vi "Apply Read Write BitField Mask.vi"(8 "error in":errorcluster, 10 "mask":enum16{"Disable", "Enable"}(ring), 11 "bitfields in":u32 format="%.0b") -> (0 "error out":errorcluster, 3 "bitfields out":u32 format="%.0b")   [LabVIEW 2020, in "Routing and Faulting Scripting.lvlib"]
uses:
  Routing and Faulting Scripting.lvlib
  NationalInstruments.VeriStand.SystemDefinitionAPI
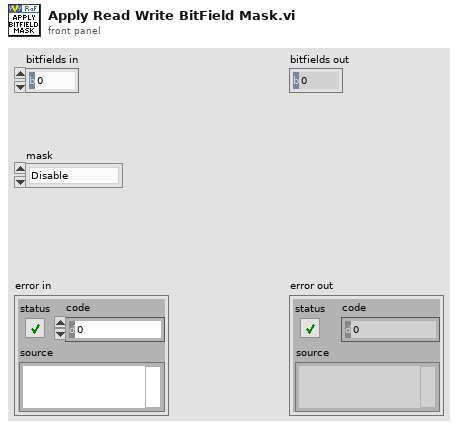
[diagram p1: front panel]
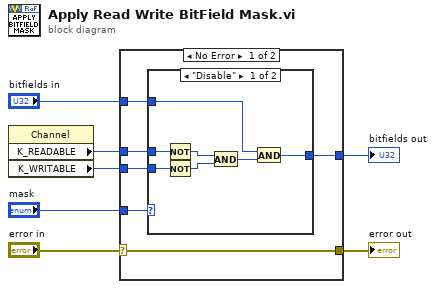
[diagram p0: block diagram]
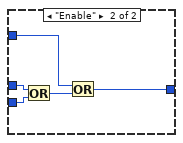
[diagram p2: hidden frame]
diagram:
  n1 = property class="Channel"() -> ("K_READABLE"=w6:u32, "K_WRITABLE"=w5:u32)  [unwired: 2 in, 2 out]
  n2 = case shown="No Error" "error in" {
    selector: "error in" -> [w8 w27]
    tunnel: "mask" -> [w13 _]
    tunnel: w6 -> [w12 _]
    tunnel: w5 -> [w11 _]
    tunnel: "bitfields in" -> [w10 w26]
    tunnel: [w9 w26] -> w3
    tunnel: [w8 w27] -> w1
    frame No Error {
      n3 = case shown="\"Disable\"" w13 {
        tunnel: w12 -> [w20 w25]
        tunnel: w11 -> [w19 w24]
        tunnel: w10 -> [w15 w23]
        tunnel: [w14 w21] -> w9
        frame "Disable" {
          n4 = Not(x=w20) -> (.not. x?=w17:u32)
          n5 = Not(x=w19) -> (.not. x?=w18:u32)
          n6 = And(x=w17, y=w18) -> (x .and. y?=w16:u32)
          n7 = And(x=w15, y=w16) -> (x .and. y?=w14:u32)
        }
        frame "Enable" {
          n8 = Or(x=w25, y=w24) -> (x .or. y?=w22:u32)
          n9 = Or(x=w23, y=w22) -> (x .or. y?=w21:u32)
        }
      }
    }
    frame Error {
    }
  }
  "bitfields out" <- w3
  "error out" <- w1
